vi "Convert Desired Position to Angle Values for Rhino.vi"(0 "Desired Position":dbl(slide)=30.0 scale=-5.0..30.0) -> (1 "Rhino at max position?":bool, 2 "Output":dbl)   [LabVIEW 2018]
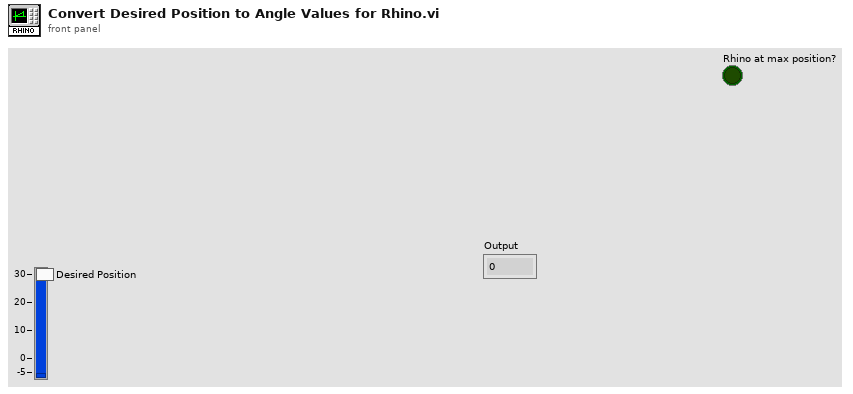
[diagram p1: front panel]
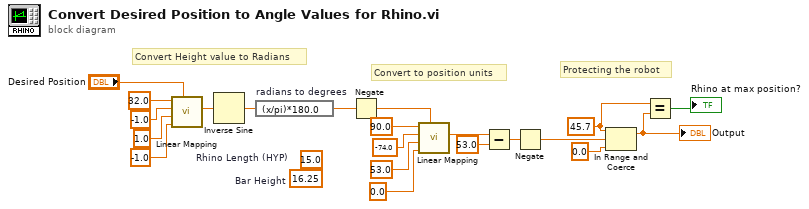
[diagram p0: block diagram]
diagram:
  w3 = 45.7 ("upper limit")
  (unwired) 16.25  # Bar Height
  (unwired) 15.0  # Rhino Length (HYP)
  # "Protecting the robot"
  # "Convert to position units"
  # "Convert Height value to Radians"
  n1 = call "Linear Mapping.vi"("X"="Desired Position", "Min B"=-1.0, "Max B"=1.0, "Min A"=-1.0, "Max A"=32.0) -> ("Y"=w21:dbl)  [unwired: 6 in]
  n2 = Inverse Sine(1:w21) -> (0:w20:dbl)
  n3 = expression code="(x/pi)*180.0" "radians to degrees"(w20) -> (w13:dbl)
  n4 = Negate(x=w13) -> (-x=w12:dbl)
  n5 = call "Linear Mapping.vi"("X"=w12, "Min B"=0.0, "Max B"=53.0, "Min A"=-74.0, "Max A"=90.0) -> ("Y"=w9:dbl)  [unwired: 6 in]
  n6 = Subtract(x=w9, y=53.0) -> (x-y=w8:dbl)
  n7 = Negate(x=w8) -> (-x=w6:dbl)
  n8 = In Range and Coerce(upper limit=w3, x=w6, lower limit=0.0) -> (coerced(x)=w2:dbl)  [unwired: 1 out]
  "Output" <- w2
  n9 = Equal?(x=w3, y=w2) -> (x = y?=→"Rhino at max position?":bool)
